vi "Create PUBLISH Packet (Client).vi"(4 "RETAIN":bool, 5 "PUBLISH type":refnum<class "PUBLISH.lvclass">, 6 "QoS":T1, 7 "DUP (Re-delivery attempt)":bool, 8 "error in (no error)":errorcluster, 9 "Packet ID (empty: generate new)":u16 format="%04x", 10 "Payload":u8[](array[numeric]) format="%08b", 11 "Topic Name":string) -> (0 "error out":errorcluster, 1 "Packet ID":u16 format="%04x", 2 "Bytes Stream":u8[](array[numeric]) format="%08b", 3 "PUBLISH":refnum<class "PUBLISH.lvclass">)   [LabVIEW 2013, in "MQTT_Control_Packets.lvlib" / "PUBLISH.lvclass"]
uses:
  PUBLISH.lvclass
  ControlPacket/QualityOfService -- enum.ctl
  ControlPacket/ControlPacket.lvclass
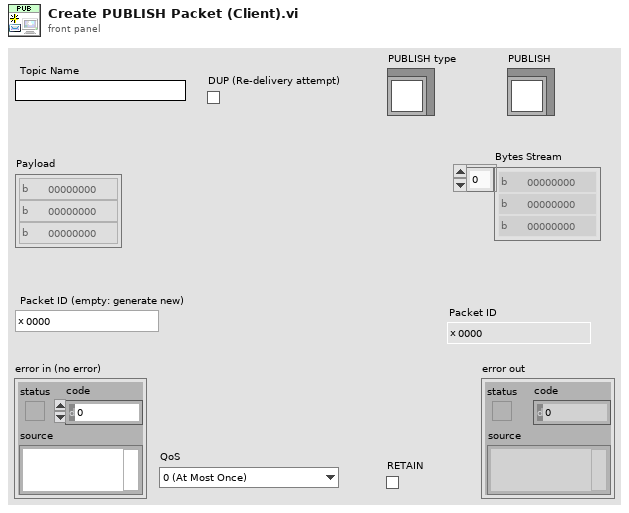
[diagram p1: front panel]
types:
  T1 = typedef "MQTT_Control_Packets.lvlib/ControlPacket.lvclass/QualityOfService -- enum.ctl" = enum16{"0 (At Most Once)", "1 (At Least Once)", "2 (Exactly Once)"}
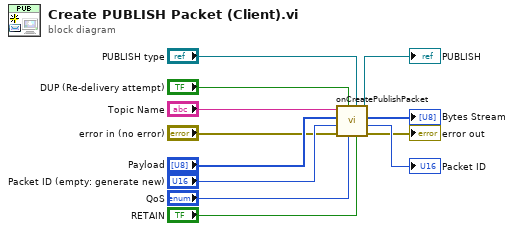
[diagram p0: block diagram]
diagram:
  n1 = call "onCreatePublishPacket.vi"("RETAIN"="RETAIN", "PUBLISH type"="PUBLISH type", "QoS"="QoS", "DUP (Re-delivery attempt)"="DUP (Re-delivery attempt)", "error in (no error)"="error in (no error)", "Packet ID (empty: generate new)"="Packet ID (empty: generate new)", "Payload"="Payload", "Topic Name"="Topic Name") -> ("error out"=→"error out":errorcluster, "Packet ID"=→"Packet ID":u16, "Bytes Stream"=→"Bytes Stream":u8[], "PUBLISH"=→"PUBLISH":refnum<class "PUBLISH.lvclass">)
